vi "Highlight Address.vi"(10 "Address":u16 format="%04x", 11 "Hex Viewer in":refnum<class "Hex Viewer.lvclass">) -> ()   [LabVIEW 2021, in "Hex Viewer.lvclass"]
uses:
  Hex Viewer.lvclass
  Hex Viewer.lvclass/Hex Viewer.ctl
  <vilib>/Utility/miscctls.llb/LVRowAndColumnTypeDef.ctl
  <vilib>/Utility/miscctls.llb/LVRowAndColumnUnsignedTypeDef.ctl
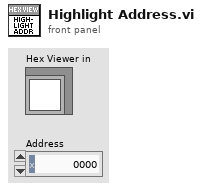
[diagram p1: front panel]
types:
  T1 = typedef "LVRowAndColumnUnsignedTypeDef.ctl" = cluster{"Row":u32, "Column":u32}
  T2 = typedef "LVRowAndColumnTypeDef.ctl" = cluster{"Row":i32, "Column":i32}
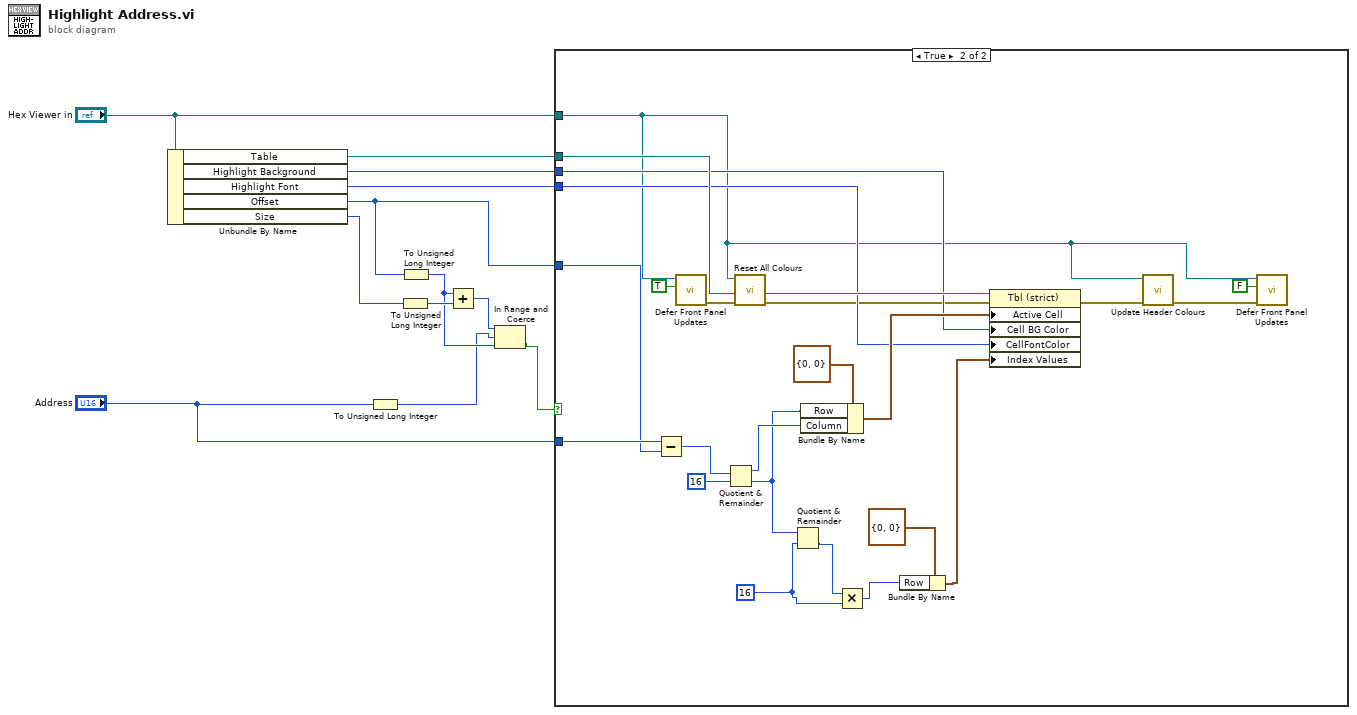
[diagram p0: block diagram]
diagram:
  n1 = Unbundle By Name("Hex Viewer in") -> ("Table"=w12:refnum<vi>, "Highlight Background"=w11:u32, "Highlight Font"=w10:u32, "Offset"=w6:u16, "Size"=w5:u16)
  n2 = To Unsigned Long Integer(number="Address") -> (unsigned 32bit integer=w1:u32)
  n3 = To Unsigned Long Integer(number=w5) -> (unsigned 32bit integer=w4:u32)
  n4 = To Unsigned Long Integer(number=w6) -> (unsigned 32bit integer=w3:u32)
  n5 = Add(x=w3, y=w4) -> (x+y=w8:u32)
  n6 = In Range and Coerce(upper limit=w8, x=w1, lower limit=w3) -> (In Range?=w7:bool)  [unwired: 1 out]
  n7 = case shown="True" w7 {
    tunnel: w12 -> [_ w35]
    tunnel: w11 -> [_ w32]
    tunnel: w10 -> [_ w31]
    tunnel: "Address" -> [_ w15]
    tunnel: w6 -> [_ w14]
    tunnel: "Hex Viewer in" -> [_ w13]
    frame False {
    }
    frame True {
      w17 = u16 16 ("y")
      n8 = Subtract(x=w15, y=w14) -> (x-y=w20:u16)
      n9 = call "Defer Front Panel Updates.vi"("Defer"=TRUE, "Hex Viewer in"=w13) -> ("error out"=w28:errorcluster)  [unwired: 9 in]
      n10 = Quotient & Remainder(x=w20, y=u16 16) -> (x-y*floor(x/y)=w19:u16, floor(x/y)=w18:u16)
      n11 = call "Reset All Colours.vi"("error in (no error)"=w28, "Hex Viewer in"=w13) -> ("error out"=w30:errorcluster)  [unwired: 9 in]
      n12 = Quotient & Remainder(x=w18, y=w17) -> (floor(x/y)=w16:u16)  [unwired: 1 out]
      n13 = Bundle By Name(cluster=T2 {"Row"=0, "Column"=0} ("Active Cell:Active Cell"), "Row"=w18, "Column"=w19) -> (w33:T2)
      n14 = Multiply(x=w16, y=w17) -> (x*y=w21:u16)
      n15 = Bundle By Name(cluster=T1 {"Row"=0, "Column"=0} ("Index Values"), "Row"=w21) -> (w23:T1)
      n16 = property class="Tbl (strict)"(reference=w35, error in=w30, "Active Cell"=w33, "Cell BG Color"=w32, "CellFontColor"=w31, "Index Values"=w23) -> (error out=w26:errorcluster)  [unwired: 1 out]
      n17 = call "Update Header Colours.vi"("error in (no error)"=w26, "Hex Viewer in"=w13) -> ("error out"=w25:errorcluster)  [unwired: 9 in]
      n18 = call "Defer Front Panel Updates.vi"("error in (no error)"=w25, "Defer"=FALSE, "Hex Viewer in"=w13) -> ()  [unwired: 8 in, 1 out]
    }
  }
